vi "ReadDIs.vi"(8 "error in":errorcluster, 10 "Digital Inputs":T1, 11 "VISA resource name":refnum<visa-resource-name>) -> (0 "error out":errorcluster, 2 "DI Status":bool, 3 "VISA resource name out":refnum<visa-resource-name>)   [LabVIEW 2020, in "HandsOnPi2040.lvlib"]
uses:
  HandsOnPi2040.lvlib
  DigIns.ctl
  <vilib>/CTI/CTI Visa Drivers/CTI-Visa/CTI-Visa.lvlib
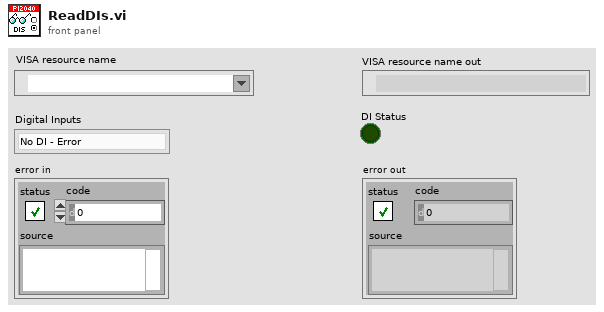
[diagram p1: front panel]
types:
  T1 = typedef "HandsOnPi2040.lvlib/DigIns.ctl" = enum16{"No DI - Error", "DI1 (GPIO7)", "DI2 (GPIO8)", "DI3 (GPIO9)", "DI4 (GPIO10)"}
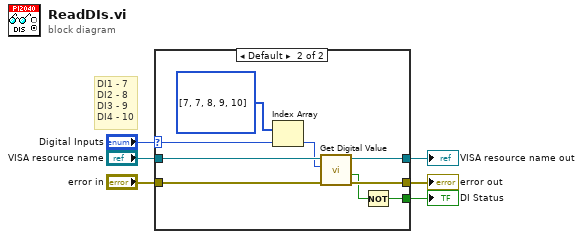
[diagram p0: block diagram]
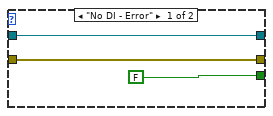
[diagram p2: hidden frame]
diagram:
  # "DI1 - 7\nDI2 - 8\nDI3 - 9\nDI4 - 10"
  n1 = case shown="Default" "Digital Inputs" {
    selector: "Digital Inputs" -> [_ w12]
    tunnel: "VISA resource name" -> [w8 w14]
    tunnel: "error in" -> [w9 w17]
    tunnel: [w8 w16] -> w4
    tunnel: [w9 w18] -> w5
    tunnel: [FALSE w10] -> w1
    frame "No DI - Error" {
    }
    frame Default {
      n2 = Index Array(array=i32[] [7, 7, 8, 9, 10], index=w12) -> (element=w13:i32)
      n3 = call <vilib>:"Get Digital Value.vi"("error in (no error)"=w17, "Channel"=w13, "VISA resource name in"=w14) -> ("error out"=w18:errorcluster, "Value"=w15:bool, "VISA resource name"=w16:refnum<visa-resource-name>)  [unwired: 6 in]
      n4 = Not(x=w15) -> (.not. x?=w10:bool)
    }
  }
  "VISA resource name out" <- w4
  "DI Status" <- w1
  "error out" <- w5
